vi "Command Handler.vi"(8 "error in (no error)":errorcluster, 10 "Dispatcher Command":T4={"Command"=enum."Rx", "Command Parameters"={"arg1"=0, "arg2"=0}}, 11 "Dispatcher in":refnum<class "Dispatcher.lvclass">) -> (0 "error out":errorcluster, 2 "Dispatcher Response":T1, 3 "Dispatcher out":refnum<class "Dispatcher.lvclass">)   [LabVIEW 2017, in "DSF Core.lvlib" / "Dispatcher.lvclass"]
uses:
  Dispatcher.lvclass
  Interfaces/Dispatcher/Response.ctl
  Interfaces/Dispatcher/Dispatcher Interface.lvclass
  Interfaces/Dispatcher/Response Parameters.ctl
  Interfaces/Dispatcher/Response Data.ctl
  Interfaces/Dispatcher/Command.ctl
  Interfaces/Dispatcher/Command Parameters.ctl
  Interfaces/Dispatcher/Command Data.ctl
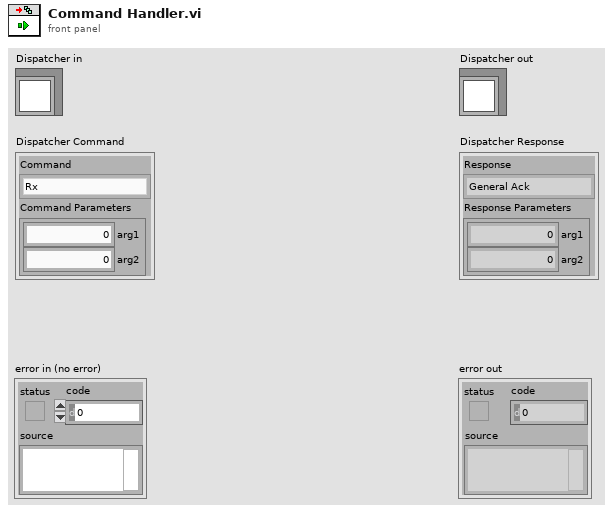
[diagram p1: front panel]
types:
  T1 = typedef "DSF Core.lvlib/Dispatcher Interface.lvclass/Response Data.ctl" = cluster{"Response":T2, "Response Parameters":T3}
  T2 = typedef "DSF Core.lvlib/Dispatcher Interface.lvclass/Response.ctl" = enum8{"General Ack", "Error", "Shutting Down"}
  T3 = typedef "DSF Core.lvlib/Dispatcher Interface.lvclass/Response Parameters.ctl" = cluster{"arg1":u64, "arg2":u64}
  T4 = typedef "DSF Core.lvlib/Dispatcher Interface.lvclass/Command Data.ctl" = cluster{"Command":T5, "Command Parameters":T6}
  T5 = typedef "DSF Core.lvlib/Dispatcher Interface.lvclass/Command.ctl" = enum8{"Offset Inline Buffers", "Rx", "Tx", "Shutdown"}
  T6 = typedef "DSF Core.lvlib/Dispatcher Interface.lvclass/Command Parameters.ctl" = cluster{"arg1":u64, "arg2":u64}
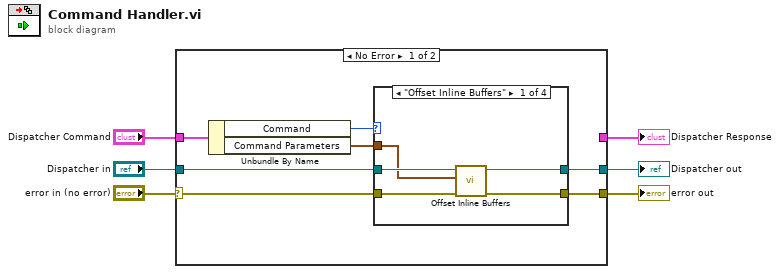
[diagram p0: block diagram]
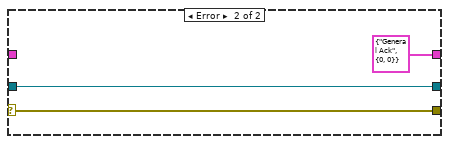
[diagram p5: hidden frame]
diagram:
  n1 = case shown="No Error" "error in (no error)" {
    selector: "error in (no error)" -> [w7 w27]
    tunnel: "Dispatcher Command" -> [w11 _]
    tunnel: "Dispatcher in" -> [w10 w26]
    tunnel: [w9 w26] -> w4
    tunnel: [w8 w27] -> w3
    tunnel: [_ T1 {"Response"=enum."General Ack", "Response Parameters"={"arg1"=0, "arg2"=0}} ("Dispatcher Response")] -> w1
    frame No Error {
      n2 = Unbundle By Name(w11) -> ("Command"=w13:T5, "Command Parameters"=w12:T6)
      n3 = case shown="\"Offset Inline Buffers\"" w13 {
        tunnel: w10 -> [w18 w20 w22 w24]
        tunnel: [w16 w20 w22 w24] -> w9
        tunnel: w7 -> [w17 w19 w21 w23]
        tunnel: [w15 w19 w21 w23] -> w8
        tunnel: w12 -> [w14 _ _ _]
        frame "Offset Inline Buffers" {
          n4 = call "Offset Inline Buffers.vi"("error in (no error)"=w17, "Command Parameters"=w14, "Dispatcher in"=w18) -> ("error out"=w15:errorcluster, "Dispatcher out"=w16:refnum<class "Dispatcher.lvclass">)  [unwired: 7 in]
        }
        frame "Rx" {
        }
        frame "Tx" {
        }
        frame "Shutdown" {
        }
      }
    }
    frame Error {
    }
  }
  "error out" <- w3
  "Dispatcher out" <- w4
  "Dispatcher Response" <- w1
